vi "limiter.vi"(2 "throttle angle":dbl, 3 "control input":dbl) -> (0 "control input limited":dbl)   [LabVIEW 2015]
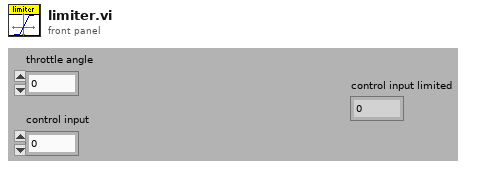
[diagram p1: front panel]
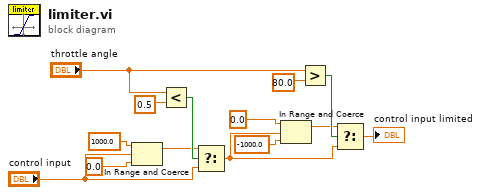
[diagram p0: block diagram]
diagram:
  n1 = In Range and Coerce(upper limit=1000.0 ("max"), x="control input", lower limit=0.0 ("min")) -> (coerced(x)=w5:dbl)  [unwired: 1 out]
  n2 = Less?(x="throttle angle", y=0.5) -> (x < y?=w13:bool)
  n3 = Select(t=w5, s=w13, f="control input") -> (s? t:f=w1:dbl)
  n4 = In Range and Coerce(upper limit=0.0 ("max"), x=w1, lower limit=-1000.0 ("min")) -> (coerced(x)=w2:dbl)  [unwired: 1 out]
  n5 = Greater?(x="throttle angle", y=80.0) -> (0:w11:bool)
  n6 = Select(t=w2, s=w11, f=w1) -> (s? t:f=→"control input limited":dbl)
